vi "extScanGlobalVarsWrite.vi"(0 "WriteDevSet":bool, 10 "scanDevTimeout(10ns)":i32, 11 "scanDevSet":bool) -> ()   [LabVIEW 2014]
uses:
  <vilib>/rvi/Emulation/niFpgaSctlEmulationGetInTimedLoop.vi
  extScanGlobalVars.vi
  <vilib>/rvi/Emulation/niFpgaProcessEmulError.vi
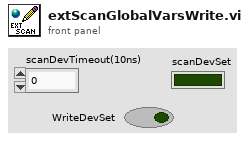
[diagram p1: front panel]
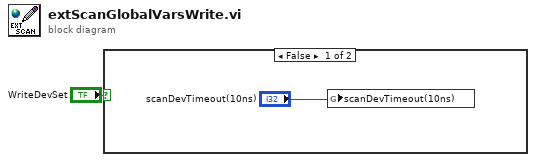
[diagram p0: block diagram]
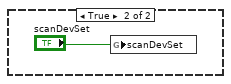
[diagram p2: hidden frame]
diagram:
  n1 = case shown="False" "WriteDevSet" {
    frame False {
      n2 = global write "extScanGlobalVars.vi" "scanDevTimeout(10ns)"("scanDevTimeout(10ns)") -> ()
    }
    frame True {
      n3 = global write "extScanGlobalVars.vi" "scanDevSet"("scanDevSet") -> ()
    }
  }
